vi "PostScanAction.vi"(0 "Device en entrée":refnum<class "EGG5210.lvclass"> caption="DNL_LabVIEW Object in", 5 "AcqComp":bool, 7 "ScanDev":bool caption="AcqComp", 11 "error in (no error)":errorcluster caption="entrée d'erreur (pas d'erreur)") -> (4 "Device en sortie":refnum<class "EGG5210.lvclass"> caption="DNL_LabVIEW Object out", 6 "PostScanString":string, 15 "error out":errorcluster caption="sortie d'erreur")   [LabVIEW 2019, in "EGG5210.lvclass"]
uses:
  EGG5210.lvclass
  C:/Programmes Labview/LabscanV1A/DevicesClass/BaseDevice/BaseDevice.lvclass
  EGG5210.lvclass/EGG5210.ctl
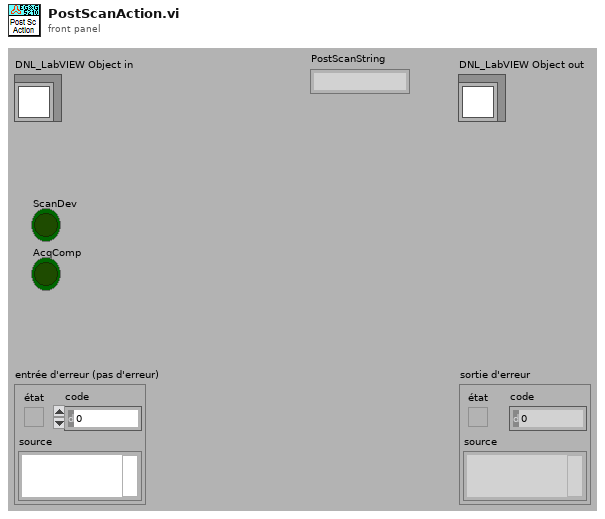
[diagram p1: front panel]
types:
  T1 = typedef "EGG5210.lvclass/EGG5210_Func.ctl" = enum16{"Read X & Y (V)", "Read Mag & Phase (V,°)", "Read X, Y, Mag & Phase (V,V,V,°)", "Read ADC Ch1 (V)", "Read ADC Ch2 (V)", "Oscillator Ctrl (Hz, mV rms)", "PL Excimer Settings (Na)"}
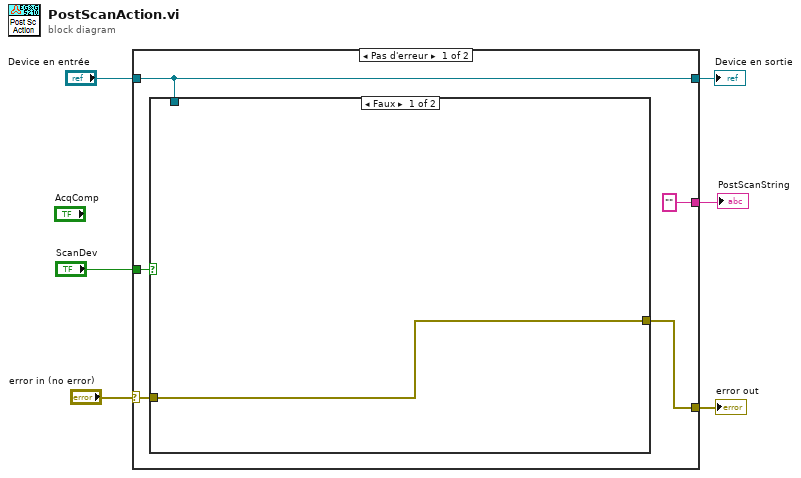
[diagram p0: block diagram]
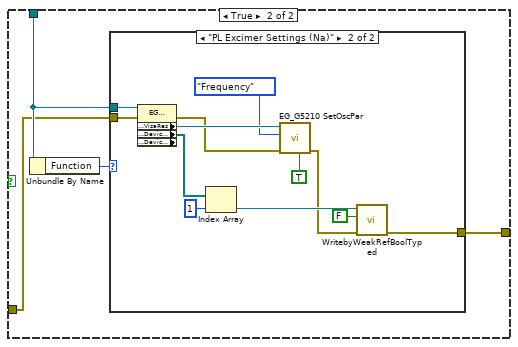
[diagram p2: hidden frame]
diagram:
  n1 = case shown="Pas d'erreur" "error in (no error)" {
    selector: "error in (no error)" -> [w10 w30]
    tunnel: [w11 w31] -> w5
    tunnel: "Device en entrée" -> [w11 w31]
    tunnel: [w9 w30] -> w3
    tunnel: ["" _] -> w2
    tunnel: "ScanDev" -> [w7 _]
    frame No Error {
      n2 = case shown="Faux" w7 {
        tunnel: w11 -> [_ w15]
        tunnel: w10 -> [w12 w14]
        tunnel: [w12 w13] -> w9
        frame False {
        }
        frame True {
          n3 = Unbundle By Name(w15) -> ("Function"=w16:T1)
          n4 = case shown="\"PL Excimer Settings (Na)\"" w16 {
            tunnel: w15 -> [_ w29]
            tunnel: w14 -> [w17 w27]
            tunnel: [w17 w19] -> w13
            frame "Read X & Y (V)", Default {
            }
            frame "PL Excimer Settings (Na)" {
              n5 = property class="EGG5210.lvclass" props=["Accessor:VisaRes", "Accessor:DeviceCtrl", "Accessor:DeviceCtrl"](reference=w29, error in=w27) -> (error out=w26:errorcluster, "Accessor:VisaRes"=w28:refnum<visa-resource-name>, "Accessor:DeviceCtrl"=w24:refnum<vi>[])  [unwired: 2 out]
              n6 = Index Array(array=w24, index=1 ("indice")) -> (element=w22:refnum<vi>)
              n7 = call <userlib>:"EG_G5210 SetOscPar.vi"("Disable Osc"=TRUE, "error in (no error)"=w26, "Énum"=enum16{"Amplitude", "Frequency"}."Frequency", "Ressource VISA"=w28) -> ("error out"=w20:errorcluster)  [unwired: 6 in, 1 out]
              n8 = call <userlib>:"WritebyWeakRefBoolTyped.vi"("error in"=w20, "Valeur"=FALSE, "Control Ref"=w22) -> ("error out"=w19:errorcluster)  [unwired: 8 in]
            }
          }
        }
      }
    }
    frame Error {
    }
  }
  "error out" <- w3
  "Device en sortie" <- w5
  "PostScanString" <- w2
